vi "Establish Connection.vi"(8 "error in":errorcluster, 9 "Caller's Queue In":refnum<class "DQMH-GenNet Message Queue.lvclass">, 10 "Module ID":i32, 11 "Data Cluster":T1) -> (0 "error out":errorcluster, 3 "Data Cluster out":T1)   [LabVIEW 2014, in "GenNet-Client.lvlib"]
doc: "Opens the TCP/IP connection to the GenNet Server module and evaluates the result. \n\nThe connection parameters are stored in this module's data cluster for potential (re)connection attempts."
uses:
  GenNet-Client.lvlib
  Module Data--cluster.ctl
  DQMH-GenNet Message Queue.lvclass
  <vilib>/Utility/error.llb/Clear Errors.vi
  hse-gennet.lvlib
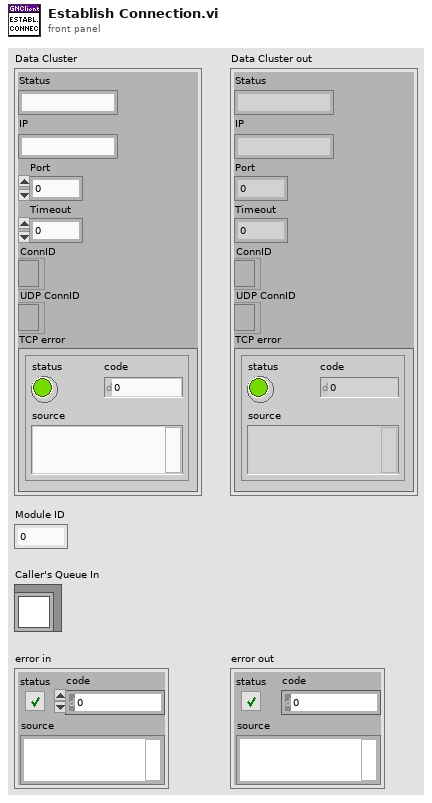
[diagram p1: front panel]
types:
  T1 = typedef "GenNet-Client.lvlib/Module Data--cluster.ctl" = cluster{"Status":string, "IP":string, "Port":u16, "Timeout":i32, "ConnID":refnum<k5>, "UDP ConnID":refnum<k16>, "TCP error":errorcluster}
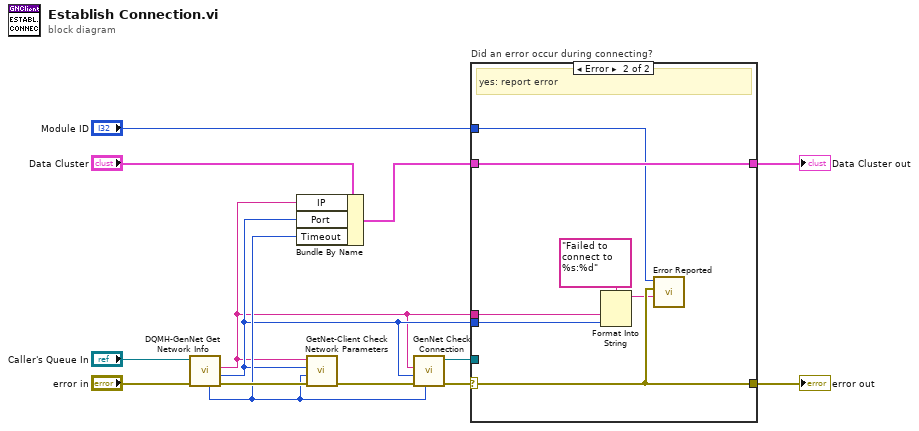
[diagram p0: block diagram]
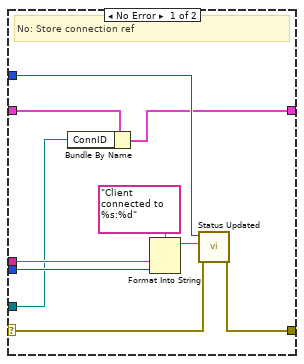
[diagram p2: hidden frame]
diagram:
  n1 = call "DQMH-GenNet Get Network Info.vi"("error in (no error)"="error in", "Message Queue in"="Caller's Queue In") -> ("error out"=w12:errorcluster, "Port Number"=w8:u16, "IP Address"=w7:string, "Timeout"=w10:i32)  [unwired: 5 in, 1 out]
  n2 = Bundle By Name(cluster="Data Cluster", "IP"=w7, "Port"=w8, "Timeout"=w10) -> (w6:T1)
  n3 = call "GetNet-Client Check Network Parameters.vi"("error in (no error)"=w12, "Timeout"=w10, "Port"=w8, "IP"=w7) -> ("error out"=w13:errorcluster)  [unwired: 7 in]
  n4 = call "GenNet Check Connection.vi"("timeout [ms]"=w10, "error in (no error)"=w13, "remote port"=w8, "ip address"=w7) -> ("error out"=w9:errorcluster, "TCP Network Connection out"=w4:refnum<k5>)  [unwired: 6 in]
  n5 = case "Did an error occur during connecting?" shown="Error" w9 {
    selector: w9 -> [w17 w26]
    tunnel: "Module ID" -> [w23 w30]
    tunnel: w4 -> [w18 _]
    tunnel: w7 -> [w22 w28]
    tunnel: w8 -> [w21 w27]
    tunnel: [w15 w26] -> w2
    tunnel: [w19 w31] -> w3
    tunnel: w6 -> [w20 w31]
    frame No Error {
      # "No: Store connection ref"
      n6 = Bundle By Name(cluster=w20, "ConnID"=w18) -> (w19:T1)
      n7 = Format Into String(format string="Client connected to %s:%d", w22, w21) -> (resulting string=w16:string)  [unwired: 2 in, 1 out]
      n8 = call "Status Updated.vi"("error in (no error)"=w17, "Status"=w16, "Module ID"=w23) -> ("error out"=w15:errorcluster)  [unwired: 8 in]
    }
    frame Error {
      # "yes: report error"
      n9 = Format Into String(format string="Failed to connect to %s:%d", w28, w27) -> (resulting string=w25:string)  [unwired: 2 in, 1 out]
      n10 = call "Error Reported.vi"("Additional Information"=w25, "Error"=w26, "Module ID"=w30) -> ()  [unwired: 8 in, 1 out]
    }
  }
  "Data Cluster out" <- w3
  "error out" <- w2
